vi "NNPC_Save.vi"(6 "Save_Options":T1, 7 "Dst Folder":path=path "D/Ngene/Projects_SVN/DeepLTK/R_and_D/Patchcore/LabVIEW/Coresets/2024_05_03/Experiments/Test", 8 "error in":errorcluster, 11 "PCore_Instance in":T2 {"NN out"."LR_Update_Policy"."WarmUp_Ratio" min=1; "NN out"."LR_Update_Policy"."WarmUp_Iter" min=1; "NN out"."LR_Update_Policy"."LR0" format="%.7f"; "Dataset_Stats"."vars"."R" format="%#_3g"; "Dataset_Stats"."vars"."G" format="%#_3g"; "Dataset_Stats"."vars"."B" format="%#_3g"; "Dataset_Stats"."means"."R" format="%#_3g"; "Dataset_Stats"."means"."G" format="%#_3g"; "Dataset_Stats"."means"."B" format="%#_3g"}) -> (0 "error out":errorcluster, 2 "Generated Files":path[](array[path]), 3 "PCore_Instance out":T2 {"NN out"."LR_Update_Policy"."WarmUp_Ratio" min=1; "NN out"."LR_Update_Policy"."WarmUp_Iter" min=1; "NN out"."LR_Update_Policy"."LR0" format="%.7f"; "Dataset_Stats"."vars"."R" format="%#_3g"; "Dataset_Stats"."vars"."G" format="%#_3g"; "Dataset_Stats"."vars"."B" format="%#_3g"; "Dataset_Stats"."means"."R" format="%#_3g"; "Dataset_Stats"."means"."G" format="%#_3g"; "Dataset_Stats"."means"."B" format="%#_3g"})   [LabVIEW 2020]
uses:
  Controls/PatchCore_Instance.ctl
  Controls/PatchCore_DS_Stats.ctl
  Controls/Image_Stats_RGB.ctl
  <vilib>/Ngene/Deep Learning Toolkit/Toolkit/NN_Network/Controls/NN.ctl
  <vilib>/Ngene/Deep Learning Toolkit/Toolkit/NN_Layers/Controls/NN_Layer_ref.ctl
  <vilib>/Ngene/Deep Learning Toolkit/Toolkit/NN_Layers/Controls/NN_Layer.ctl
  <vilib>/Ngene/Deep Learning Toolkit/Toolkit/NN_Layers/Controls/NN_Layer_Type.ctl
  <vilib>/Ngene/Deep Learning Toolkit/Toolkit/NN_Data/API/NN_Dims(C,H,W).ctl
  <vilib>/Ngene/Deep Learning Toolkit/Toolkit/NN_Layers/Controls/NN_Layer_Metrics.ctl
  <vilib>/Ngene/Deep Learning Toolkit/Toolkit/NN_Network/Controls/NN_Device.ctl
  <vilib>/Ngene/Deep Learning Toolkit/Toolkit/NNg/cuda/Controls/nng_cuda_handles.ctl
  <vilib>/Ngene/Deep Learning Toolkit/Toolkit/NN_Layers/Controls/NN_Layer_Dimty.ctl
  <vilib>/Ngene/Deep Learning Toolkit/Toolkit/NN_Layers/Controls/NN_Layer_RF_State.ctl
  <vilib>/Ngene/Deep Learning Toolkit/Toolkit/NN_Data/API/NN_Dims(V,H).ctl
  <vilib>/Ngene/Deep Learning Toolkit/Toolkit/NN_Network/Controls/NN_In_Out_Dim-ty.ctl
  <vilib>/Ngene/Deep Learning Toolkit/Toolkit/NN_Train/Controls/NN_Train_Params.ctl
  <vilib>/Ngene/Deep Learning Toolkit/Toolkit/NN_Train/Controls/NN_Train_Optimizer.ctl
  <vilib>/Ngene/Deep Learning Toolkit/Toolkit/NN_Train/Controls/NN_Train_Data_Sampling.ctl
  <vilib>/Ngene/Deep Learning Toolkit/Toolkit/NN_Train/Controls/NN_LR_Policy_Cfg.ctl
  <vilib>/Ngene/Deep Learning Toolkit/Toolkit/NN_Train/Controls/NN_LR_Policy_Type.ctl
  <vilib>/Ngene/Deep Learning Toolkit/Toolkit/NN_Train/Controls/NN_Train_Session_Data.ctl
  <vilib>/Ngene/Deep Learning Toolkit/Toolkit/NN_Data/Controls/NN_Ground_truth.ctl
  <vilib>/Ngene/Deep Learning Toolkit/Toolkit/NN_Train/Controls/NN_Loss_Type.ctl
  <vilib>/Ngene/Deep Learning Toolkit/Toolkit/NNg/Network/WS/Controls/NNG_WS.ctl
  <vilib>/Ngene/Deep Learning Toolkit/Toolkit/NNg/Network/WS/Controls/NNg_WS_Mem_DVR.ctl
  <vilib>/Ngene/Deep Learning Toolkit/Toolkit/NNg/cuda/Controls/cuda_Mem_desc.ctl
  Controls/PCore_Device.ctl
  Controls/PatchCore_Init_CFG.ctl
  Controls/PatchCore_BackBone_Selector.ctl
  Controls/Coreset_Params.ctl
  Controls/Random_Projection_Coreset.ctl
  Controls/MemBank_and_Norm_Variants.ctl
  Controls/Model_Saving_Params.ctl
  <vilib>/Ngene/CuLab - GPU Accelerated Toolkit/Toolkit/Low_Level/Tensor_Classes/T_Children/T2D/T2D_Children/T2D_SGL/T2D_SGL.lvclass
  <vilib>/Ngene/CuLab - GPU Accelerated Toolkit/Toolkit/Low_Level/Tensor_Classes/T_Children/T2D/T2D_Children/T2D_SGL/Pull.vi
  <vilib>/Ngene/CuLab - GPU Accelerated Toolkit/Toolkit/CuLab.lvlib
  <vilib>/Ngene/Deep Learning Toolkit/Toolkit/Deep_Learning_Toolkit_by_Ngene.lvlib
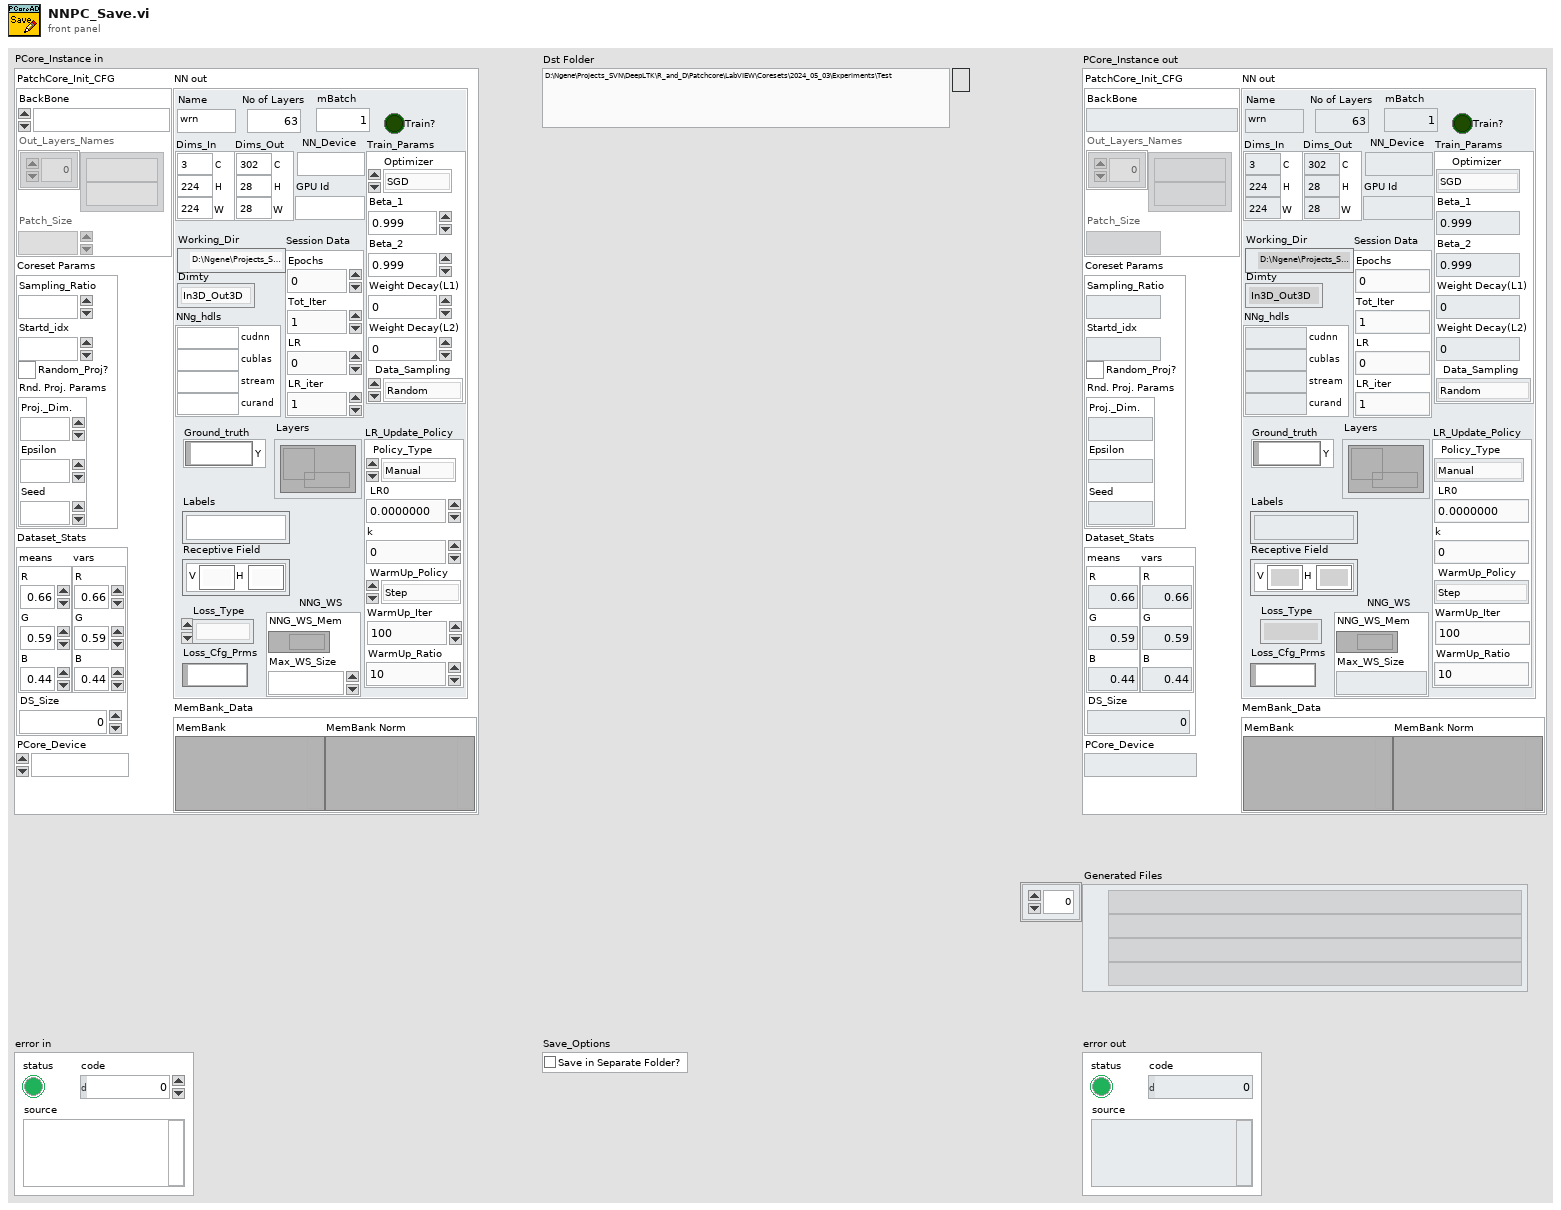
[diagram p1: front panel]
types:
  T1 = typedef "Model_Saving_Params.ctl" = cluster{"Save in Separate Folder?":bool}
  T2 = typedef "PatchCore_Instance.ctl" = cluster{"Dataset_Stats":T3, "NN":T5, "PCore_Device":T22, "PatchCore_Init_CFG":T23, "Coreset Params":T25, "MemBank_Data":T27}
  T3 = typedef "PatchCore_DS_Stats.ctl" = cluster{"means":T4, "vars":T4, "DS_Size":i32}
  T4 = typedef "Image_Stats_RGB.ctl" = cluster{"R":sgl, "G":sgl, "B":sgl}
  T5 = typedef "Deep_Learning_Toolkit_by_Ngene.lvlib/NN.ctl" = cluster{"Name":string, "No of Layers":i32, "mBatch":i32, "Layers":T6[], "Dimty":T7, "Dims_In":T8, "Dims_Out":T8, "Working_Dir":path, "Train?":bool, "Train_Params":T9, "LR_Update_Policy":T12, "Session Data":T14, "Ground_truth":T15, "NNg_hdls":T16, "NN_Device":T17, "GPU Id":i32, "Labels":string[], "Receptive Field":T18[], "Loss_Type":T19, "Loss_Cfg_Prms":variant, "NNG_WS":T20}
  T6 = typedef "Deep_Learning_Toolkit_by_Ngene.lvlib/NN_Layer_ref.ctl" = refnum<data-value>
  T7 = typedef "Deep_Learning_Toolkit_by_Ngene.lvlib/NN_In_Out_Dim-ty.ctl" = enum8{"In1D_Out1D", "In3D_Out1D", "In3D_Out3D", "In3D_OutBBox"}
  T8 = typedef "Deep_Learning_Toolkit_by_Ngene.lvlib/NN_Dims(C,H,W).ctl" = cluster{"C":i32, "H":i32, "W":i32}
  T9 = typedef "Deep_Learning_Toolkit_by_Ngene.lvlib/NN_Train_Params.ctl" = cluster{"Optimizer":T10, "Beta_1":sgl, "Beta_2":sgl, "Weight Decay(L1)":sgl, "Weight Decay(L2)":sgl, "Data_Sampling":T11}
  T10 = typedef "Deep_Learning_Toolkit_by_Ngene.lvlib/NN_Train_Optimizer.ctl" = enum16{"SGD", "Adam", "Adagrad", "Adadelta", "RMSProp", "Nesterov"}
  T11 = typedef "Deep_Learning_Toolkit_by_Ngene.lvlib/NN_Train_Data_Sampling.ctl" = enum16{"Random", "Sequential"}
  T12 = typedef "Deep_Learning_Toolkit_by_Ngene.lvlib/NN_LR_Policy_Cfg.ctl" = cluster{"Policy_Type":T13, "LR0":dbl, "k":sgl, "WarmUp_Policy":enum16{"Step", "Ramp"}, "WarmUp_Iter":i32, "WarmUp_Ratio":sgl}
  T13 = typedef "Deep_Learning_Toolkit_by_Ngene.lvlib/NN_LR_Policy_Type.ctl" = enum16{"Manual", "Step", "Exp", "1/t"}
  T14 = typedef "Deep_Learning_Toolkit_by_Ngene.lvlib/NN_Train_Session_Data.ctl" = cluster{"Epochs":sgl, "Tot_Iter":i32, "LR":sgl, "LR_iter":i32}
  T15 = typedef "Deep_Learning_Toolkit_by_Ngene.lvlib/NN_Ground_truth.ctl" = cluster{"Y":variant}
  T16 = typedef "Deep_Learning_Toolkit_by_Ngene.lvlib/nng_cuda_handles.ctl" = cluster{"cudnn":u64, "cublas":u64, "stream":u64, "curand":u64}
  T17 = typedef "Deep_Learning_Toolkit_by_Ngene.lvlib/NN_Device.ctl" = enum16{"CPU", "GPU"}
  T18 = typedef "Deep_Learning_Toolkit_by_Ngene.lvlib/NN_Dims(V,H).ctl" = cluster{"V":i32, "H":i32}
  T19 = typedef "Deep_Learning_Toolkit_by_Ngene.lvlib/NN_Loss_Type.ctl" = enum16{"None", "MSE", "CrossEntropy", "YOLO_v2", "YOLO_v4"}
  T20 = typedef "Deep_Learning_Toolkit_by_Ngene.lvlib/NNG_WS.ctl" = cluster{"NNG_WS_Mem":T21, "Max_WS_Size":i64}
  T21 = typedef "Deep_Learning_Toolkit_by_Ngene.lvlib/NNg_WS_Mem_DVR.ctl" = refnum<data-value>
  T22 = typedef "PCore_Device.ctl" = enum16{"CPU", "GPU(CuLab)"}
  T23 = typedef "PatchCore_Init_CFG.ctl" = cluster{"BackBone":T24, "Out_Layers_Names":string[], "Patch_Size":u32}
  T24 = typedef "PatchCore_BackBone_Selector.ctl" = enum16{"WRN_50_2_L2L3"}
  T25 = typedef "Coreset_Params.ctl" = cluster{"Sampling_Ratio":sgl, "Startd_idx":i32, "Random_Proj?":bool, "Rnd. Proj. Params":T26}
  T26 = typedef "Random_Projection_Coreset.ctl" = cluster{"Proj._Dim.":i32, "Epsilon":sgl, "Seed":i32}
  T27 = typedef "MemBank_and_Norm_Variants.ctl" = cluster{"MemBank":variant, "MemBank Norm":variant}
  T28 = enum16{"open", "replace", "create", "open or create", "replace or create", "replace or create with confirmation"}
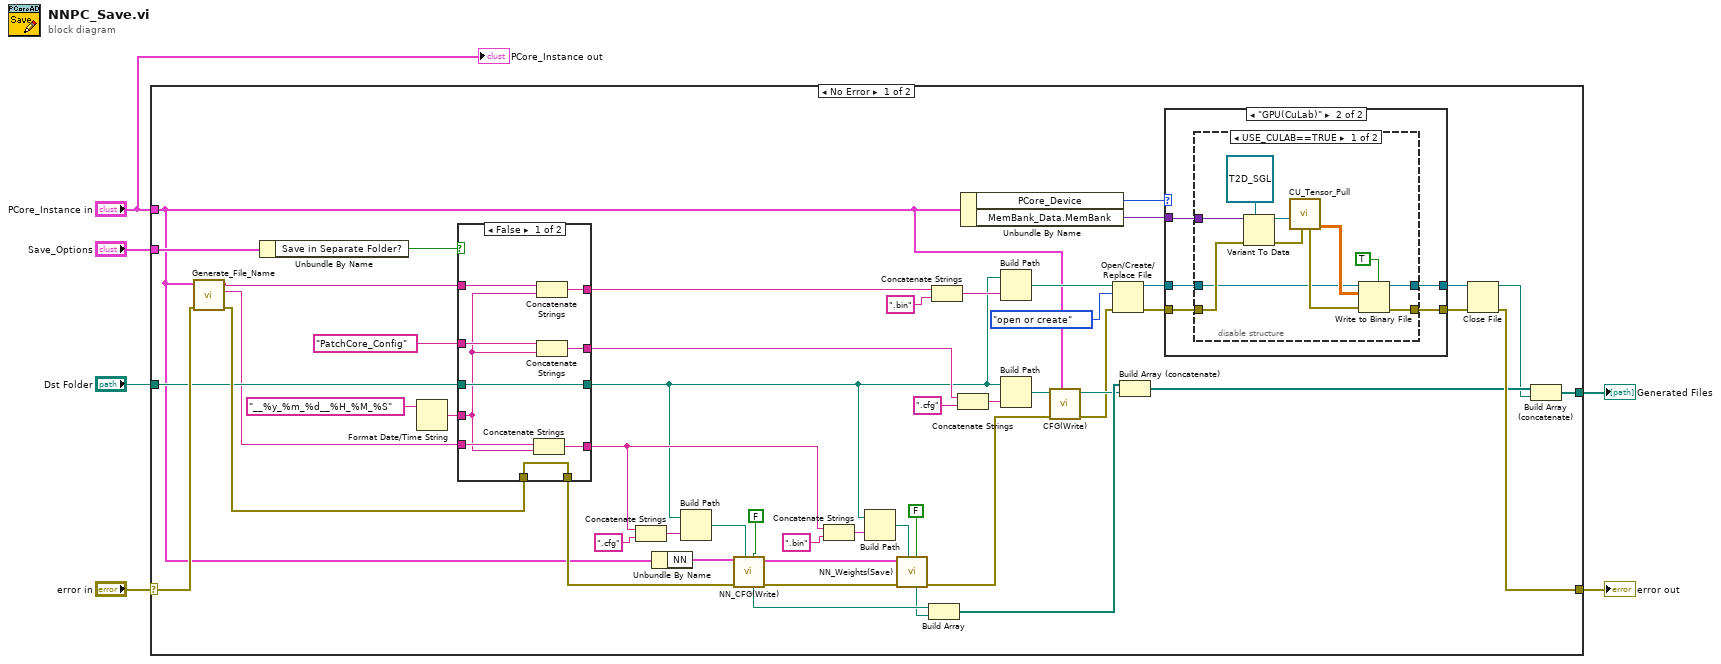
[diagram p0: block diagram]
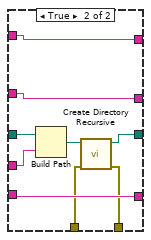
[diagram p2: hidden frame]
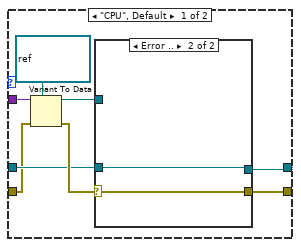
[diagram p3: hidden frame]
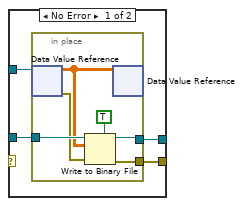
[diagram p4: hidden frame]
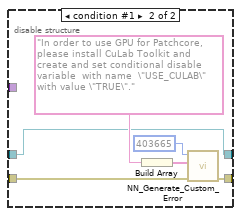
[diagram p5: hidden frame]
diagram:
  n1 = case shown="No Error" "error in" {
    selector: "error in" -> [w56 w117]
    tunnel: "Dst Folder" -> [w15 _]
    tunnel: "PCore_Instance in" -> [w8 _]
    tunnel: [w51 w117] -> w5
    tunnel: [w49 _] -> w3
    tunnel: "Save_Options" -> [w53 _]
    frame No Error {
      n2 = call "Generate_File_Name.vi"("error in"=w56, "PCore_Instance in"=w8) -> ("error out"=w55:errorcluster, "NN_Model_Name"=w10:string, "Patchcore_Name"=w11:string)  [unwired: 7 in]
      n3 = Unbundle By Name(w53) -> ("Save in Separate Folder?"=w52:bool)
      n4 = Format Date/Time String(time format string (%c)="__%y_%m_%d__%H_%M_%S") -> (date/time string=w13:string)  [unwired: 2 in]
      n5 = case shown="False" w52 {
        tunnel: w10 -> [w65 w72]
        tunnel: w11 -> [w63 w73]
        tunnel: [w64 w72] -> w47
        tunnel: [w62 w73] -> w45
        tunnel: [w61 w74] -> w46
        tunnel: "PatchCore_Config" ("string") -> [w60 w74]
        tunnel: [w59 w68] -> w9
        tunnel: w15 -> [w59 w71]
        tunnel: w13 -> [w58 w70]
        tunnel: w55 -> [w57 w67]
        tunnel: [w57 w66] -> w12
        frame False {
          n6 = Concatenate Strings(w65, w58) -> (w64:string)
          n7 = Concatenate Strings(w63, w58) -> (w62:string)
          n8 = Concatenate Strings(w60, w58) -> (w61:string)
        }
        frame True {
          n9 = Build Path(base path=w71, name or relative path=w70) -> (appended path=w69:path)
          n10 = call <vilib>:"Create Directory Recursive.vi"("error in (no error)"=w67, "directory"=w69) -> ("error out"=w66:errorcluster, "directory copy"=w68:path)  [unwired: 3 in, 1 out]
        }
      }
      n11 = Concatenate Strings(w47, ".cfg" ("string")) -> (w23:string)
      n12 = Unbundle By Name(w8) -> ("NN"=w28:T5)
      n13 = Build Path(base path=w9, name or relative path=w23) -> (appended path=w22:path)
      n14 = call <vilib>:"NN_CFG(Write).vi"("Append Timestamp? (T)"=FALSE, "CFG Save path"=w22, "error in (no error)"=w12, "NN in"=w28) -> ("error out"=w26:errorcluster, "NN out"=w27:T5, "CFG File Path"=w19:path)  [unwired: 5 in]
      n15 = Concatenate Strings(w47, ".bin" ("string")) -> (w21:string)
      n16 = Build Path(base path=w9, name or relative path=w21) -> (appended path=w20:path)
      n17 = call <vilib>:"NN_Weights(Save).vi"("Append Timestamp? (T)"=FALSE, "Weight Save Path"=w20, "error in (no error)"=w26, "NN in"=w27) -> ("error out"=w54:errorcluster, "Weight Path out"=w18:path)  [unwired: 5 in, 1 out]
      n18 = Build Array(w19, w18) -> (w50:path[])
      n19 = Concatenate Strings(w45, ".bin" ("string")) -> (w44:string)
      n20 = Concatenate Strings(w46, ".cfg" ("string")) -> (w39:string)
      n21 = Unbundle By Name(w8) -> ("PCore_Device"=w29:T22, "MemBank_Data.MemBank"=w34:variant)
      n22 = Build Path(base path=w9, name or relative path=w44) -> (appended path=w43:path)
      n23 = Build Path(base path=w9, name or relative path=w39) -> (appended path=w38:path)
      n24 = call "CFG(Write).vi"("PCore_Instance"=w8, "error in (no error)"=w54, "CFG File Path"=w38) -> ("error out"=w36:errorcluster, "CFG File Path"=w37:path)  [unwired: 7 in]
      n25 = Open/Create/Replace File(file path (use dialog)=w43, error in=w36, operation (0:open)=T28."open or create") -> (refnum out=w35:refnum<file>, error out=w33:errorcluster)  [unwired: 3 in, 1 out]
      n26 = Build Array (concatenate)(w50, w37) -> (w41:path[])
      n27 = case shown="\"GPU(CuLab)\"" w29 {
        tunnel: [w75 w99] -> w30
        tunnel: [w76 w98] -> w31
        tunnel: w35 -> [w79 w95]
        tunnel: w34 -> [w78 w97]
        tunnel: w33 -> [w77 w96]
        frame "CPU", Default {
          n28 = Variant To Data(error in=w77, type=refnum<data-value> refnum ("MemBank DVR"), Variant=w78) -> (data=w81:refnum<data-value>, error out=w80:errorcluster)
          n29 = case shown="Error .." w80 {
            selector: w80 -> [_ w94]
            tunnel: [w86 w93] -> w76
            tunnel: [w85 w94] -> w75
            tunnel: w79 -> [w84 w93]
            tunnel: w81 -> [w83 _]
            frame No Error {
              n30 = in-place {
                in-place-border: w84 -> [w92]
                in-place-border: [w90] -> w86
                in-place-border: [w88] -> w85
                n31 = in-place-dvr #1(w83) -> (w91:sgl[][], w87:errorcluster)
                n32 = Write to Binary File(file (use dialog)=w92, data=w91, error in=w87, 5:TRUE ("prepend array or string size? (T)")) -> (refnum out=w90:refnum<file>, error out=w88:errorcluster)  [unwired: 2 in, 1 out]
                n33 = in-place-dvr #1(w91) -> ()  [unwired: 2 out]
              }
            }
            frame Error {
            }
          }
        }
        frame "GPU(CuLab)" {
          n34 = disable-structure shown="USE_CULAB==TRUE" {
            disable-tunnel: [w108 w113] -> w99
            disable-tunnel: [w100 w111] -> w98
            disable-tunnel: w97 -> [w103 _]
            disable-tunnel: w96 -> [w102 w112]
            disable-tunnel: w95 -> [w101 w111]
            frame condition #0 (active) {
              n35 = Variant To Data(error in=w102, type=refnum<class "T2D_SGL.lvclass"> refnum ("MemBank DVR"), Variant=w103) -> (data=w106:refnum<class "T2D_SGL.lvclass">, error out=w105:errorcluster)
              n36 = call-poly <vilib>:"CU_Tensor_Pull.vi"("error in (no error)"=w105, "T2D_SGL in"=w106) -> ("2D_SGL_Data"=w109:sgl[][], "error out"=w104:errorcluster)  [unwired: 7 in, 1 out]
              n37 = Write to Binary File(file (use dialog)=w101, data=w109, error in=w104, 5:TRUE ("prepend array or string size? (T)")) -> (refnum out=w100:refnum<file>, error out=w108:errorcluster)  [unwired: 2 in, 1 out]
            }
            frame condition #1 {
              n38 = Build Array("In order to use GPU for Patchcore, please install CuLab Toolkit and create and set conditional disable variable  with name  \"USE_CULAB\" with value \"TRUE\"." ("Message")) -> (w115:string[])
              n39 = call <vilib>:"NN_Generate_Custom_Error.vi"("error in (no error)"=w112, "Message"=w115, "Error_code"=403665) -> ("error out"=w113:errorcluster)  [unwired: 8 in]
            }
          }
        }
      }
      n40 = Close File(refnum=w31, error in=w30) -> (path=w32:path, error out=w51:errorcluster)
      n41 = Build Array (concatenate)(w41, w32) -> (w49:path[])
    }
    frame Error {
    }
  }
  "error out" <- w5
  "Generated Files" <- w3
  "PCore_Instance out" <- "PCore_Instance in"
